vi "Get_Joystick.vi"(1 "Joystick_One":string="Pilot Controller", 2 "Joystick_Two":string="CoPilot Controller") -> (6 "Joystick_Out":T1)   [LabVIEW 2020]
uses:
  <vilib>/Rock Robotics/WPI/Joystick/WPI_JoystickDeviceEnum.ctl
  Joystick_Controls.ctl
panel:
  in  "Joystick Controls":T1
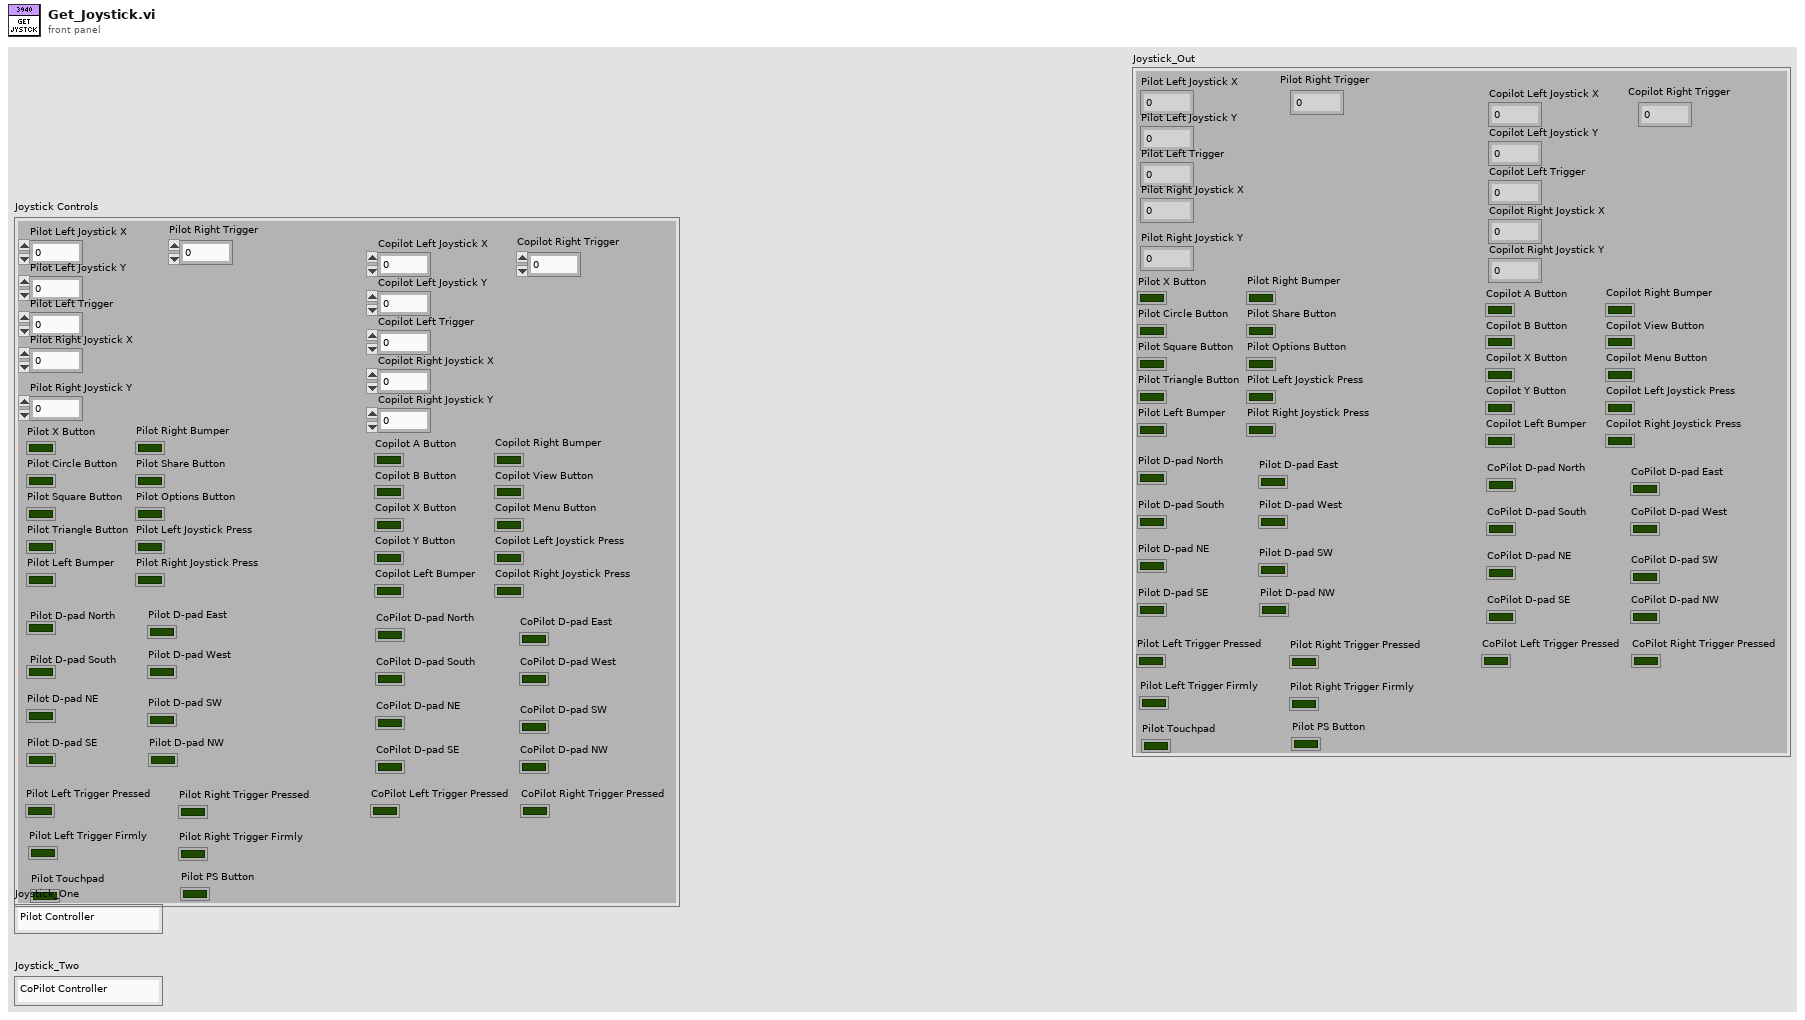
[diagram p1: front panel]
types:
  T1 = typedef "Joystick_Controls.ctl" = cluster{"Pilot Left Joystick X":dbl, "Pilot Left Joystick Y":dbl, "Pilot X Button":bool, "Pilot Circle Button":bool, "Pilot Square Button":bool, "Pilot Triangle Button":bool, "Pilot Left Bumper":bool, "Pilot Right Bumper":bool, "Pilot Share Button":bool, "Pilot Options Button":bool, "Pilot Left Joystick Press":bool, "Pilot Right Joystick Press":bool, "Pilot Left Trigger":dbl, "Pilot Right Joystick X":dbl, "Pilot Right Joystick Y":dbl, "Pilot Right Trigger":dbl, "Copilot Left Joystick X":dbl, "Copilot Left Joystick Y":dbl, "Copilot A Button":bool, "Copilot B Button":bool, "Copilot X Button":bool, "Copilot Y Button":bool, "Copilot Left Bumper":bool, "Copilot Right Bumper":bool, "Copilot View Button":bool, "Copilot Menu Button":bool, "Copilot Left Joystick Press":bool, "Copilot Right Joystick Press":bool, "Copilot Left Trigger":dbl, "Copilot Right Joystick X":dbl, "Copilot Right Joystick Y":dbl, "Copilot Right Trigger":dbl, "Pilot D-pad North":bool, "Pilot D-pad South":bool, "Pilot D-pad East":bool, "Pilot D-pad West":bool, "Pilot D-pad NE ":bool, "Pilot D-pad SE":bool, "Pilot D-pad SW":bool, "Pilot D-pad NW":bool, "CoPilot D-pad North":bool, "CoPilot D-pad South":bool, "CoPilot D-pad East":bool, "CoPilot D-pad West":bool, "CoPilot D-pad NE":bool, "CoPilot D-pad SE":bool, "CoPilot D-pad SW":bool, "CoPilot D-pad NW":bool, "Pilot Left Trigger Pressed":bool, "Pilot Right Trigger Pressed":bool, "CoPilot Left Trigger Pressed":bool, "CoPilot Right Trigger Pressed":bool, "Pilot Left Trigger Firmly":bool, "Pilot Right Trigger Firmly":bool, "Pilot Touchpad":bool, "Pilot PS Button":bool}
  T2 = typedef "WPI_JoystickDeviceEnum.ctl" = enum16{"USB 0", "USB 1", "USB 2", "USB 3", "USB 4", "USB 5"}
  T3 = typedef "WPI_Joystick Info.ctl" = cluster{"Device Name":string, "HID Type":T4, "XBox Type":T5, "Axes Count":i32, "Axes Types":T6[], "Button Count":i32, "POV Count":i32}
  T4 = typedef "WPI_JoystickHID Types.ctl" = enum16{"Not HID", "HID Joystick", "HID Gamepad", "HID Driving Wheel", "HID Flightstick", "HID First Person"}
  T5 = typedef "WPI_JoystickXBox Types.ctl" = enum16{"Not XBox", "XBox Unknown", "XBox Gamepad", "XBox Wheel", "XBox Arcade Stick", "XBox Flight Stick", "XBox Dance Pad", "XBox Guitar", "XBox Drum Kit", "XBox Arcade Pad"}
  T6 = typedef "WPI_JoystickAxis Types.ctl" = enum16{"X Axis", "Y Axis", "Z Axis", "RxAxis", "RyAxis", "RzAxis", "Slider", "POV", "None", "L X Axis", "L Y Axis", "L Trigger", "R Trigger", "R X Axis", "R Y Axis"}
  T7 = typedef "WPI_JoystickDevRef.ctl" = cluster{"Device":T2}
  T8 = cluster{"Axes[0]":dbl, "Axes[1]":dbl, "Axes[2]":dbl, "Axes[3]":dbl, "Axes[4]":dbl, "Axes[5]":dbl, "Axes[6]":dbl, "Axes[7]":dbl, "Axes[8]":dbl}
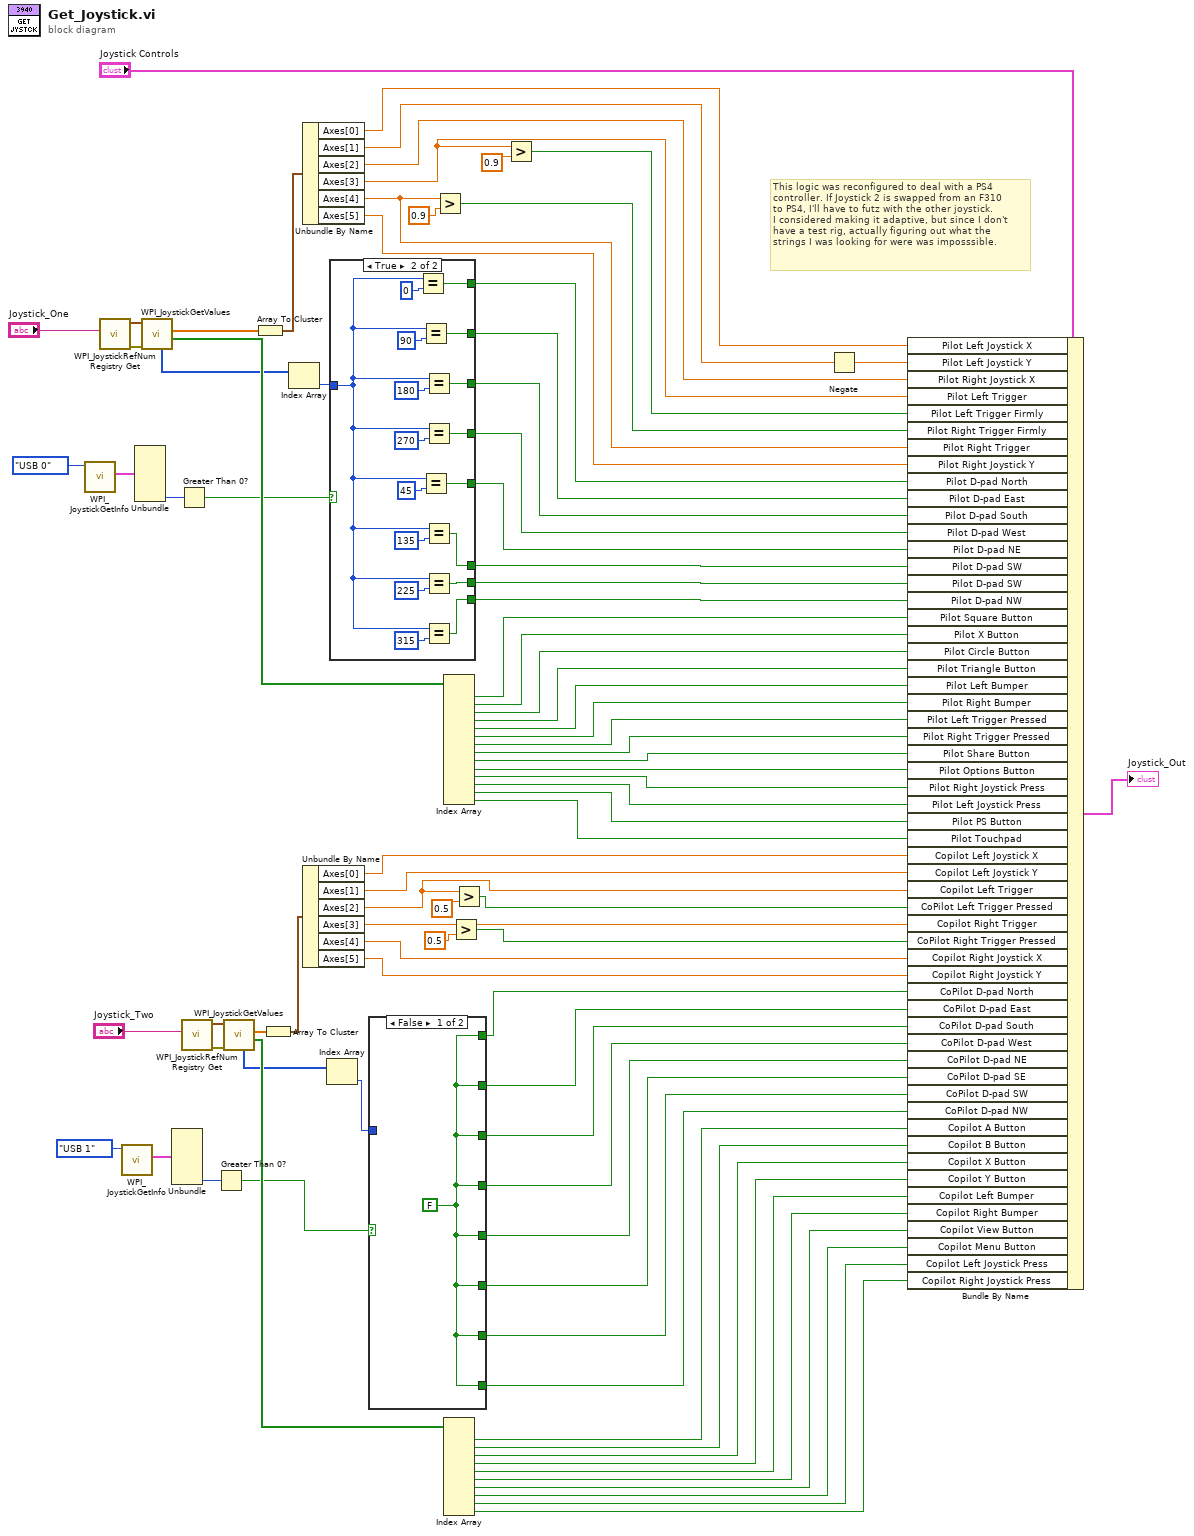
[diagram p0: block diagram]
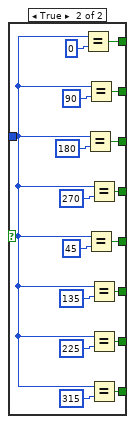
[diagram p2: hidden frame]
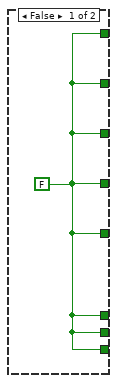
[diagram p3: hidden frame]
diagram:
  # "This logic was reconfigured to deal with a PS4\ncontroller. If Joystick 2 is swapped from an F310\nto PS4, I'll have to futz with the other joystick.\nI considered making it adaptive, but since I don't\nhave a test rig, actually figuring out what the\nstrings I was looking for were was imposssible."
  n1 = call <vilib>:"WPI_JoystickGetInfo.vi"("JoystickDevice"=WPI_JoystickDeviceEnum."USB 0") -> ("Joystick Info"=w20:T3)  [unwired: 9 in, 1 out]
  n2 = call <vilib>:"WPI_JoystickRefNum Registry Get.vi"("refnum name"="Joystick_One") -> ("error out"=w51:errorcluster, "JoystickDevRef"=w87:T7)  [unwired: 9 in]
  n3 = call <vilib>:"WPI_JoystickGetInfo.vi"("JoystickDevice"=WPI_JoystickDeviceEnum."USB 1") -> ("Joystick Info"=w16:T3)  [unwired: 9 in, 1 out]
  n4 = Unbundle(w20) -> ("POV Count"=w19:i32)  [unwired: 6 out]
  n5 = call <vilib>:"WPI_JoystickGetValues.vi"("error in (no error)"=w51, "JoystickDevRef"=w87) -> ("Buttons"=w81:bool[], "Axes"=w86:dbl[], "POVs"=w53:i16[])  [unwired: 5 in, 2 out]
  n6 = Unbundle(w16) -> ("POV Count"=w15:i32)  [unwired: 6 out]
  n7 = Greater Than 0?(x=w19) -> (x > 0?=w18:bool)
  n8 = call <vilib>:"WPI_JoystickRefNum Registry Get.vi"("refnum name"="Joystick_Two") -> ("error out"=w50:errorcluster, "JoystickDevRef"=w70:T7)  [unwired: 9 in]
  n9 = Greater Than 0?(x=w15) -> (x > 0?=w14:bool)
  n10 = call <vilib>:"WPI_JoystickGetValues.vi"("error in (no error)"=w50, "JoystickDevRef"=w70) -> ("Buttons"=w68:bool[], "Axes"=w69:dbl[], "POVs"=w52:i16[])  [unwired: 5 in, 2 out]
  n11 = Array To Cluster(array=w86) -> (cluster=w85:T8)
  n12 = Array To Cluster(array=w69) -> (cluster=w67:T8)
  n13 = Index Array(array=w53) -> (element=w40:i16)  [unwired: 1 in]
  n14 = Unbundle By Name(w85) -> ("Axes[0]"=w84:dbl, "Axes[1]"=w83:dbl, "Axes[2]"=w13:dbl, "Axes[3]"=w12:dbl, "Axes[4]"=w10:dbl, "Axes[5]"=w82:dbl)
  n15 = Unbundle By Name(w67) -> ("Axes[0]"=w7:dbl, "Axes[1]"=w6:dbl, "Axes[2]"=w29:dbl, "Axes[3]"=w26:dbl, "Axes[4]"=w66:dbl, "Axes[5]"=w65:dbl)
  n16 = Index Array(array=w52) -> (element=w32:i16)  [unwired: 1 in]
  n17 = case shown="True" w18 {
    tunnel: [w88 w105] -> w47
    tunnel: [w88 w104] -> w46
    tunnel: [w88 w103] -> w45
    tunnel: [w88 w102] -> w44
    tunnel: [w88 w101] -> w43
    tunnel: [w88 w100] -> w42
    tunnel: [w88 w99] -> w41
    tunnel: w40 -> [_ w89]
    tunnel: [w88 w90] -> w23
    frame False {
      w88 = FALSE
    }
    frame True {
      n18 = Equal?(x=w89, y=i16 0) -> (x = y?=w90:bool)
      n19 = Equal?(x=w89, y=i16 90) -> (x = y?=w105:bool)
      n20 = Equal?(x=w89, y=i16 45) -> (x = y?=w101:bool)
      n21 = Equal?(x=w89, y=i16 180) -> (x = y?=w104:bool)
      n22 = Equal?(x=w89, y=i16 270) -> (x = y?=w103:bool)
      n23 = Equal?(x=w89, y=i16 135) -> (x = y?=w100:bool)
      n24 = Equal?(x=w89, y=i16 225) -> (x = y?=w99:bool)
      n25 = Equal?(x=w89, y=i16 315) -> (x = y?=w102:bool)
    }
  }
  n26 = case shown="False" w14 {
    tunnel: [w106 w115] -> w5
    tunnel: [w106 w114] -> w39
    tunnel: [w106 w107] -> w38
    tunnel: [w106 w113] -> w37
    tunnel: [w106 w112] -> w36
    tunnel: [w106 w111] -> w35
    tunnel: [w106 w110] -> w34
    tunnel: [w106 w109] -> w33
    tunnel: w32 -> [_ w108]
    frame False {
      w106 = FALSE
    }
    frame True {
      n27 = Equal?(x=w108, y=i16 0) -> (x = y?=w115:bool)
      n28 = Equal?(x=w108, y=i16 180) -> (x = y?=w107:bool)
      n29 = Equal?(x=w108, y=i16 90) -> (x = y?=w114:bool)
      n30 = Equal?(x=w108, y=i16 45) -> (x = y?=w112:bool)
      n31 = Equal?(x=w108, y=i16 270) -> (x = y?=w113:bool)
      n32 = Equal?(x=w108, y=i16 135) -> (x = y?=w111:bool)
      n33 = Equal?(x=w108, y=i16 225) -> (x = y?=w110:bool)
      n34 = Equal?(x=w108, y=i16 315) -> (x = y?=w109:bool)
    }
  }
  n35 = Greater?(x=w10, y=0.9) -> (0:w8:bool)
  n36 = Index Array(array=w81) -> (element #1=w80:bool, element #2=w79:bool, element #3=w78:bool, element #4=w77:bool, element #5=w76:bool, element #6=w75:bool, element #7=w74:bool, element #8=w73:bool, element #9=w72:bool, element #10=w71:bool, element #11=w4:bool, element #12=w3:bool, element #13=w2:bool, element #14=w1:bool)  [unwired: 14 in]
  n37 = Index Array(array=w68) -> (element #1=w64:bool, element #2=w63:bool, element #3=w62:bool, element #4=w61:bool, element #5=w59:bool, element #6=w60:bool, element #7=w58:bool, element #8=w57:bool, element #9=w56:bool, element #10=w55:bool)  [unwired: 10 in]
  n38 = Greater?(x=w26, y=0.5) -> (0:w27:bool)
  n39 = Greater?(x=w29, y=0.5) -> (0:w30:bool)
  n40 = Greater?(x=w12, y=0.9) -> (0:w11:bool)
  n41 = Negate(x=w83) -> (-x=w22:dbl)
  n42 = Bundle By Name(cluster="Joystick Controls", "Pilot Left Joystick X"=w84, "Pilot Left Joystick Y"=w22, "Pilot Right Joystick X"=w13, "Pilot Left Trigger"=w12, "Pilot Left Trigger Firmly"=w11, "Pilot Right Trigger Firmly"=w8, "Pilot Right Trigger"=w10, "Pilot Right Joystick Y"=w82, "Pilot D-pad North"=w23, "Pilot D-pad East"=w47, "Pilot D-pad South"=w46, "Pilot D-pad West"=w45, "Pilot D-pad NE"=w43, "Pilot D-pad SW"=w42, "Pilot D-pad SW"=w41, "Pilot D-pad NW"=w44, "Pilot Square Button"=w80, "Pilot X Button"=w79, "Pilot Circle Button"=w78, "Pilot Triangle Button"=w77, "Pilot Left Bumper"=w76, "Pilot Right Bumper"=w75, "Pilot Left Trigger Pressed"=w74, "Pilot Right Trigger Pressed"=w73, "Pilot Share Button"=w72, "Pilot Options Button"=w71, "Pilot Right Joystick Press"=w4, "Pilot Left Joystick Press"=w3, "Pilot PS Button"=w2, "Pilot Touchpad"=w1, "Copilot Left Joystick X"=w7, "Copilot Left Joystick Y"=w6, "Copilot Left Trigger"=w29, "CoPilot Left Trigger Pressed"=w30, "Copilot Right Trigger"=w26, "CoPilot Right Trigger Pressed"=w27, "Copilot Right Joystick X"=w66, "Copilot Right Joystick Y"=w65, "CoPilot D-pad North"=w5, "CoPilot D-pad East"=w39, "CoPilot D-pad South"=w38, "CoPilot D-pad West"=w37, "CoPilot D-pad NE"=w36, "CoPilot D-pad SE"=w35, "CoPilot D-pad SW"=w34, "CoPilot D-pad NW"=w33, "Copilot A Button"=w64, "Copilot B Button"=w63, "Copilot X Button"=w62, "Copilot Y Button"=w61, "Copilot Left Bumper"=w59, "Copilot Right Bumper"=w60, "Copilot View Button"=w58, "Copilot Menu Button"=w57, "Copilot Left Joystick Press"=w56, "Copilot Right Joystick Press"=w55) -> (→"Joystick_Out":T1)
